vi "Image LinearMax.vi"(8 "error in (no error)":errorcluster, 10 "Optional Rectangle":i32[](array[numeric]), 11 "Image Src":T1) -> (0 "error out":errorcluster, 2 "X Max":i16[](graph), 3 "Y Max":i16[](graph))   [LabVIEW 2011]
uses:
  <vilib>/vision/Image Controls.llb/IMAQ Image.ctl
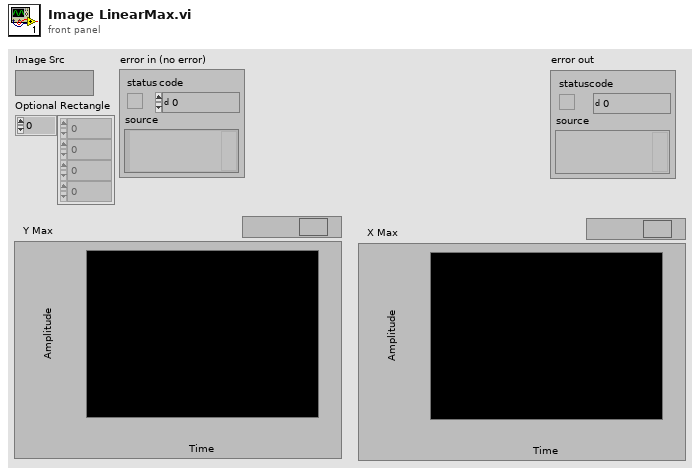
[diagram p1: front panel]
types:
  T1 = typedef "IMAQ Image.ctl" = refnum<image>
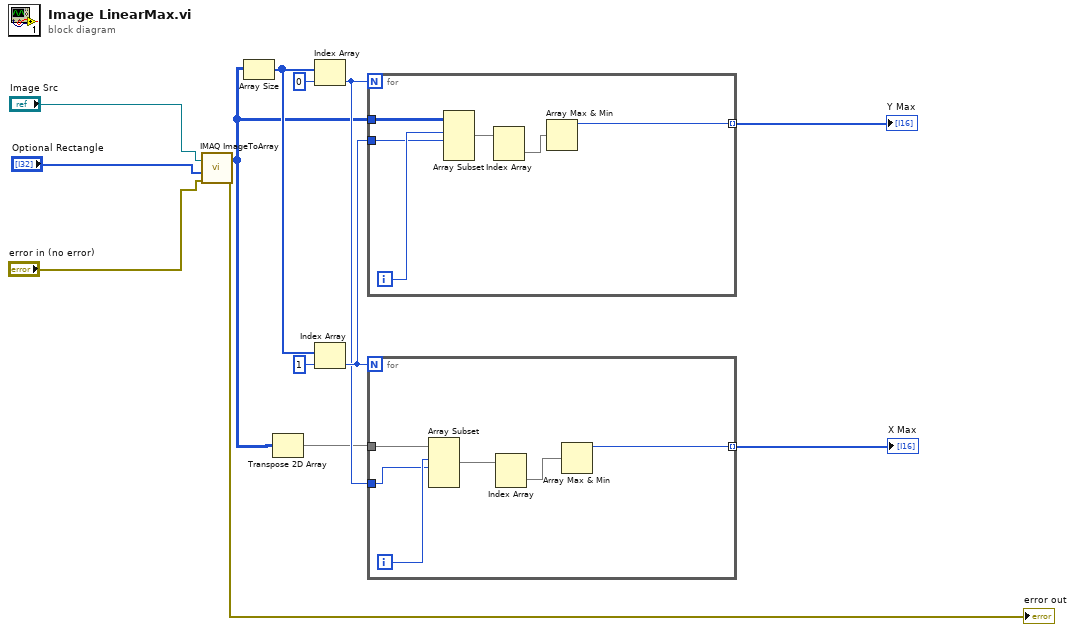
[diagram p0: block diagram]
diagram:
  n1 = call "IMAQ ImageToArray"("error in (no error)"="error in (no error)", "Optional Rectangle"="Optional Rectangle", "Image"="Image Src") -> ("error out"=→"error out":errorcluster, "Image Pixels (I16)"=w2:i16[][])  [unwired: 1 in, 3 out]
  n2 = Array Size(array=w2) -> (size(s)=w8:i32[])
  n3 = Transpose 2D Array(2D array=w2) -> (transposed array=w1:i16[][])
  n4 = Index Array(array=w8, index=0) -> (element=w6:i32)
  n5 = Index Array(array=w8, index=1) -> (element=w7:i32)
  n6 = for {
    N: w6 -> [_]
    tunnel: w2 -> [w19]
    tunnel: w7 -> [w17]
    tunnel: [w16] -> w4 mode=indexing
    i -> [w18]
    n7 = Array Subset(array=w19, index (row)=w18, length (row)=w17) -> (w15:i16[][])  [unwired: 2 in]
    n8 = Index Array(array=w15) -> (element=w14:i16[])  [unwired: 2 in]
    n9 = Array Max & Min(array=w14) -> (max value=w16:i16)  [unwired: 3 out]
  }
  "Y Max" <- w4
  n10 = for {
    N: w7 -> [_]
    tunnel: w1 -> [w25]
    tunnel: w6 -> [w20]
    tunnel: [w24] -> w3 mode=indexing
    i -> [w21]
    n11 = Array Subset(array=w25, index (row)=w21, length (row)=w20) -> (w23:i16[][])  [unwired: 2 in]
    n12 = Index Array(array=w23) -> (element=w22:i16[])  [unwired: 2 in]
    n13 = Array Max & Min(array=w22) -> (max value=w24:i16)  [unwired: 3 out]
  }
  "X Max" <- w3
